vi "AOL Z Cal-Update display msg global.vi"(11 "Motor Z":sgl) -> ()   [LabVIEW 2020]
uses:
  Globals/gl_Calibration globals.vi
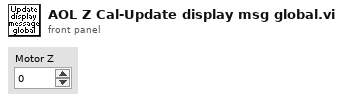
[diagram p1: front panel]
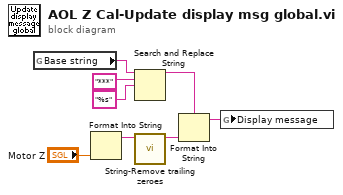
[diagram p0: block diagram]
diagram:
  n1 = global read "gl_Calibration globals.vi" "Base string"() -> (w6:string)
  n2 = Format Into String("Motor Z") -> (resulting string=w4:string)  [unwired: 3 in, 1 out]
  n3 = Search and Replace String(input string=w6, search string="***" ("format string"), replace string="%s" ("replace string (\"\")")) -> (result string=w2:string)  [unwired: 5 in, 3 out]
  n4 = call <userlib>:"String-Remove trailing zeroes.vi"("String in"=w4) -> ("String out"=w3:string)  [unwired: 10 in]
  n5 = Format Into String(format string=w2, w3) -> (resulting string=w1:string)  [unwired: 2 in, 1 out]
  n6 = global write "gl_Calibration globals.vi" "Display message"(w1) -> ()
